vi "Shooter.vi"(10 "Shooter States":T1, 11 "Shooter RPM":dbl) -> (2 "Shooter Output":dbl, 3 "Shooter at Speed?":bool)   [LabVIEW 2015]
uses:
  Typedefs/Shooter States.ctl
panel:
  in  "Disabled?":bool
  in  "I_Cap":dbl
  in  "Shot Error Thresh":dbl
  in  "Shooter Gains":cluster{"kP":dbl, "kI":dbl, "kD":dbl}
  in  "1/MaxV":dbl
  in  "Max Accel":dbl=50.0
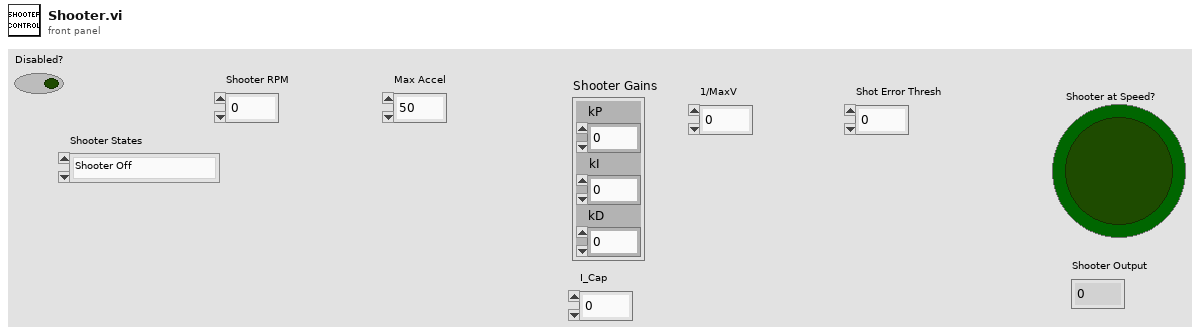
[diagram p1: front panel]
types:
  T1 = typedef "Shooter States.ctl" = enum16{"Shooter Off", "Shooter Far", "Shooter Close", "Shooter Intermediate"}
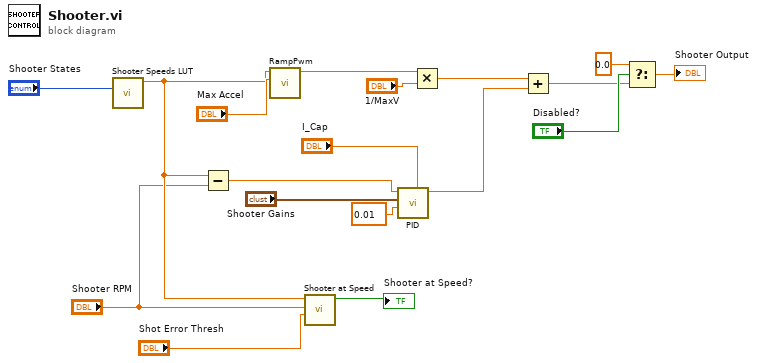
[diagram p0: block diagram]
diagram:
  n1 = call "Shooter Speeds LUT.vi"("Shooter States"="Shooter States") -> ("Target Velocity"=w3:dbl)  [unwired: 10 in]
  n2 = Subtract(x=w3, y="Shooter RPM") -> (x-y=w1:dbl)
  n3 = call "RampPwm.vi"("Ramp Step"="Max Accel", "Input"=w3) -> ("Output"=w4:dbl)  [unwired: 9 in]
  n4 = call "Shooter at Speed.vi"("Shot Error Thresh"="Shot Error Thresh", "Shooter RPM"="Shooter RPM", "Target Velocity"=w3) -> ("Shooter at Speed"=→"Shooter at Speed?":bool)  [unwired: 8 in]
  n5 = call "PID.vi"("I_Cap"="I_Cap", "Loop Period"=0.01, "Gains"="Shooter Gains", "Error"=w1) -> ("Output"=w13:dbl)  [unwired: 5 in, 2 out]
  n6 = Multiply(x=w4, y="1/MaxV") -> (x*y=w17:dbl)
  n7 = Add(x=w17, y=w13) -> (x+y=w9:dbl)
  n8 = Select(t=0.0, s="Disabled?", f=w9) -> (s? t:f=→"Shooter Output":dbl)
